vi "stream data to channel.vi"(8 "error in":errorcluster, 11 "data chunk":T1) -> (0 "error out":errorcluster)   [LabVIEW 2026, in "Nominal Core Streaming Engine.lvlib"]
uses:
  Nominal Core Streaming Engine.lvlib
  rt full channel buffer.ctl
  rt per channel buffer.ctl
  lib_nominal-streaming-lv_64.dll
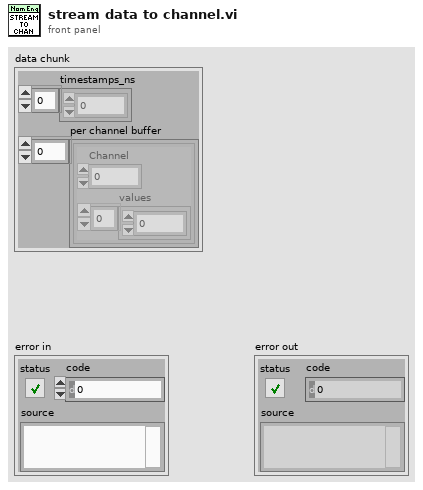
[diagram p1: front panel]
types:
  T1 = typedef "Nominal Core Streaming Engine.lvlib/rt full channel buffer.ctl" = cluster{"timestamps_ns":i64[], "per channel buffer":T2[]}
  T2 = typedef "Nominal Core Streaming Engine.lvlib/rt per channel buffer.ctl" = cluster{"Channel":u64, "values":dbl[]}
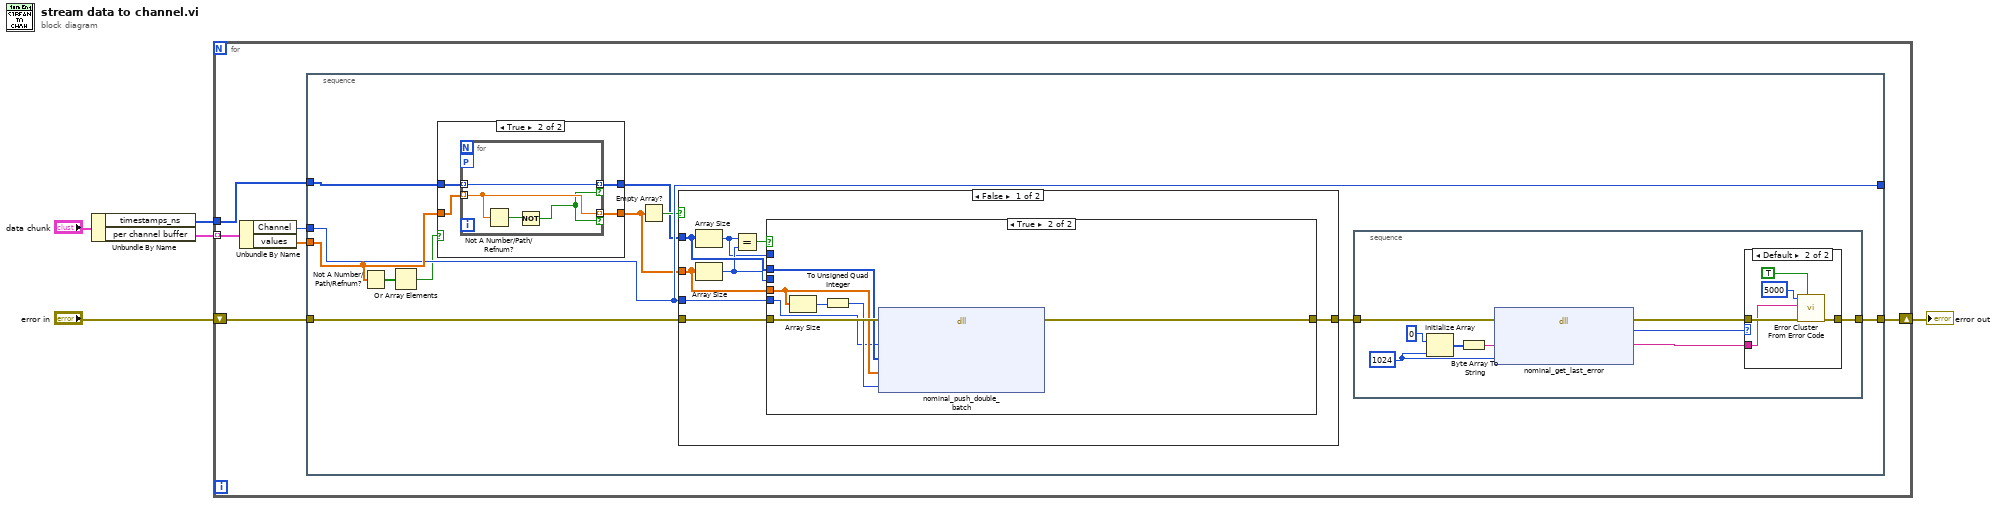
[diagram p0: block diagram]
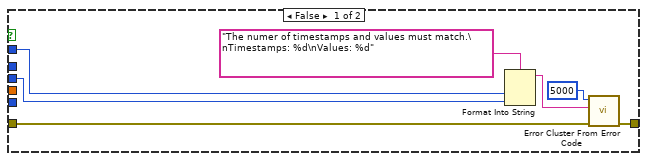
[diagram p3: hidden frame]
diagram:
  n1 = Unbundle By Name("data chunk") -> ("timestamps_ns"=w3:i64[], "per channel buffer"=w2:T2[])
  n2 = for {
    tunnel: w2 -> [w11] mode=indexing
    tunnel: w3 -> [w10]
    shift-right: [w7] -> w5
    shift-left: "error in" -> [w6]
    n3 = Unbundle By Name(w11) -> ("Channel"=w9:u64, "values"=w8:dbl[])
    n4 = stacked-sequence {
      tunnel: [w18] -> w7
      tunnel: [w17] -> _
      tunnel: w6 -> [w21]
      tunnel: w8 -> [w20]
      tunnel: w10 -> [w19]
      tunnel: w9 -> [w17]
      frame #0 {
        n5 = Not A Number/Path/Refnum?(number/path/refnum=w20) -> (NaN/Path/Refnum?=w13:bool[])
        n6 = Or Array Elements(Boolean array=w13) -> (logical OR=w12:bool)
        n7 = case shown="True" w12 {
          tunnel: w19 -> [w24 w28]
          tunnel: w20 -> [w23 w27]
          tunnel: [w24 w26] -> w14
          tunnel: [w23 w25] -> w15
          frame False {
          }
          frame True {
            n8 = for {
              tunnel: [w32] -> w26 mode=indexing if=w29
              tunnel: [w31] -> w25 mode=indexing if=w29
              workers-P: _ -> [_]
              tunnel: w28 -> [w32] mode=indexing
              tunnel: w27 -> [w31] mode=indexing
              n9 = Not A Number/Path/Refnum?(number/path/refnum=w31) -> (NaN/Path/Refnum?=w30:bool)
              n10 = Not(x=w30) -> (.not. x?=w29:bool)
            }
          }
        }
        n11 = Empty Array?(array=w15) -> (empty?=w16:bool)
        n12 = case shown="False" w16 {
          tunnel: w21 -> [w40 w55]
          tunnel: [w39 w55] -> w22
          tunnel: w14 -> [w38 _]
          tunnel: w15 -> [w37 _]
          tunnel: w17 -> [w33 _]
          frame False {
            n13 = Array Size(array=w38) -> (size(s)=w34:i32)
            n14 = Array Size(array=w37) -> (size(s)=w35:i32)
            n15 = Equal?(x=w34, y=w35) -> (x = y?=w36:bool)
            n16 = case shown="True" w36 {
              tunnel: w40 -> [w42 w53]
              tunnel: [w41 w52] -> w39
              tunnel: w38 -> [_ w50]
              tunnel: w37 -> [_ w49]
              tunnel: w35 -> [w45 _]
              tunnel: w34 -> [w44 _]
              tunnel: w33 -> [_ w48]
              frame False {
                n17 = Format Into String(format string="The numer of timestamps and values must match.\nTimestamps: %d\nValues: %d" ("error message (\"\")"), w44, w45) -> (resulting string=w43:string)  [unwired: 2 in, 1 out]
                n18 = call <vilib>:"Error Cluster From Error Code.vi"("error in (no error)"=w42, "error message (\"\")"=w43, "error code (0)"=5000) -> ("error out"=w41:errorcluster)  [unwired: 6 in]
              }
              frame True {
                n19 = Array Size(array=w49) -> (size(s)=w54:i32)
                n20 = To Unsigned Quad Integer(1:w54) -> (0:w51:u64)
                n21 = dll-call lib="C:/sw/ni-veristand-custom-device-nominal-core/source/lib_nominal-streaming-lv_*.*" fn="nominal_push_double_batch"(error in=w53, "writer_handle"=w48, "timestamps_ns"=w50, "values"=w49, "count"=w51) -> (error out=w52:errorcluster)  [unwired: 7 in, 1 out]
              }
            }
          }
          frame True {
          }
        }
        n22 = stacked-sequence {
          tunnel: [w62] -> w18
          tunnel: w22 -> [w60]
          frame #0 {
            w57 = u64 1024 ("buffer_size")
            n23 = Initialize Array(u8 0, w57) -> (w58:u8[])
            n24 = Byte Array To String(unsigned byte array=w58) -> (string=w59:string)
            n25 = dll-call lib="C:/sw/ni-veristand-custom-device-nominal-core/source/lib_nominal-streaming-lv_*.*" fn="nominal_get_last_error"(error in=w60, "buffer"=w59, "buffer_size"=w57) -> (error out=w61:errorcluster, "return type"=w64:i32, "buffer"=w63:string)  [unwired: 3 in, 1 out]
            n26 = case shown="Default" w64 {
              tunnel: w61 -> [w65 w70]
              tunnel: [w65 w69] -> w62
              tunnel: w63 -> [_ w68]
              frame -1 {
              }
              frame Default {
                n27 = call <vilib>:"Error Cluster From Error Code.vi"("show call chain? (False)"=TRUE, "error in (no error)"=w70, "error message (\"\")"=w68, "error code (0)"=5000) -> ("error out"=w69:errorcluster)  [unwired: 5 in]
              }
            }
          }
        }
      }
    }
  }
  "error out" <- w5
